vi "Add 04.vi"(1 "y":sgl, 2 "x":sgl) -> (0 "x+y":sgl)   [LabVIEW 2015]
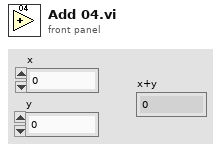
[diagram p1: front panel]
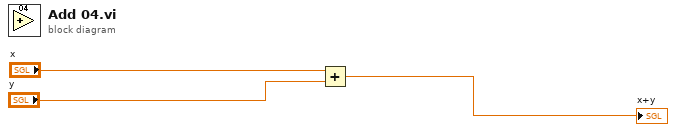
[diagram p0: block diagram]
diagram:
  n1 = Add(x="x", y="y") -> (x+y=→"x+y":sgl)
